vi "ESP_Full_State.vi"() -> ()   [LabVIEW 2021]
panel:
  in  "Channel":i32
  out "Data":dbl[](array[numeric])
  out "Stream on? UDP":string
  in  "file path 2":path
  in  "UDP Activate":bool
  out "All ESP":sgl[][](graph)
  in  "address":string="192.168.1.190"
  out "output array":sgl[][](array[numeric])
  in  "stop streaming":bool
  in  "Shut dowm":bool
  in  "Full state":bool
  in  "Stream":bool
  in  "Re-zero":bool
  out "Single ESP":sgl[](graph)
  out "Stream on?":string
  out "Full state on?":string
  out "Full state":string
  # "Sampling rate is 225 Hz, please use the Setup software to change the rate"
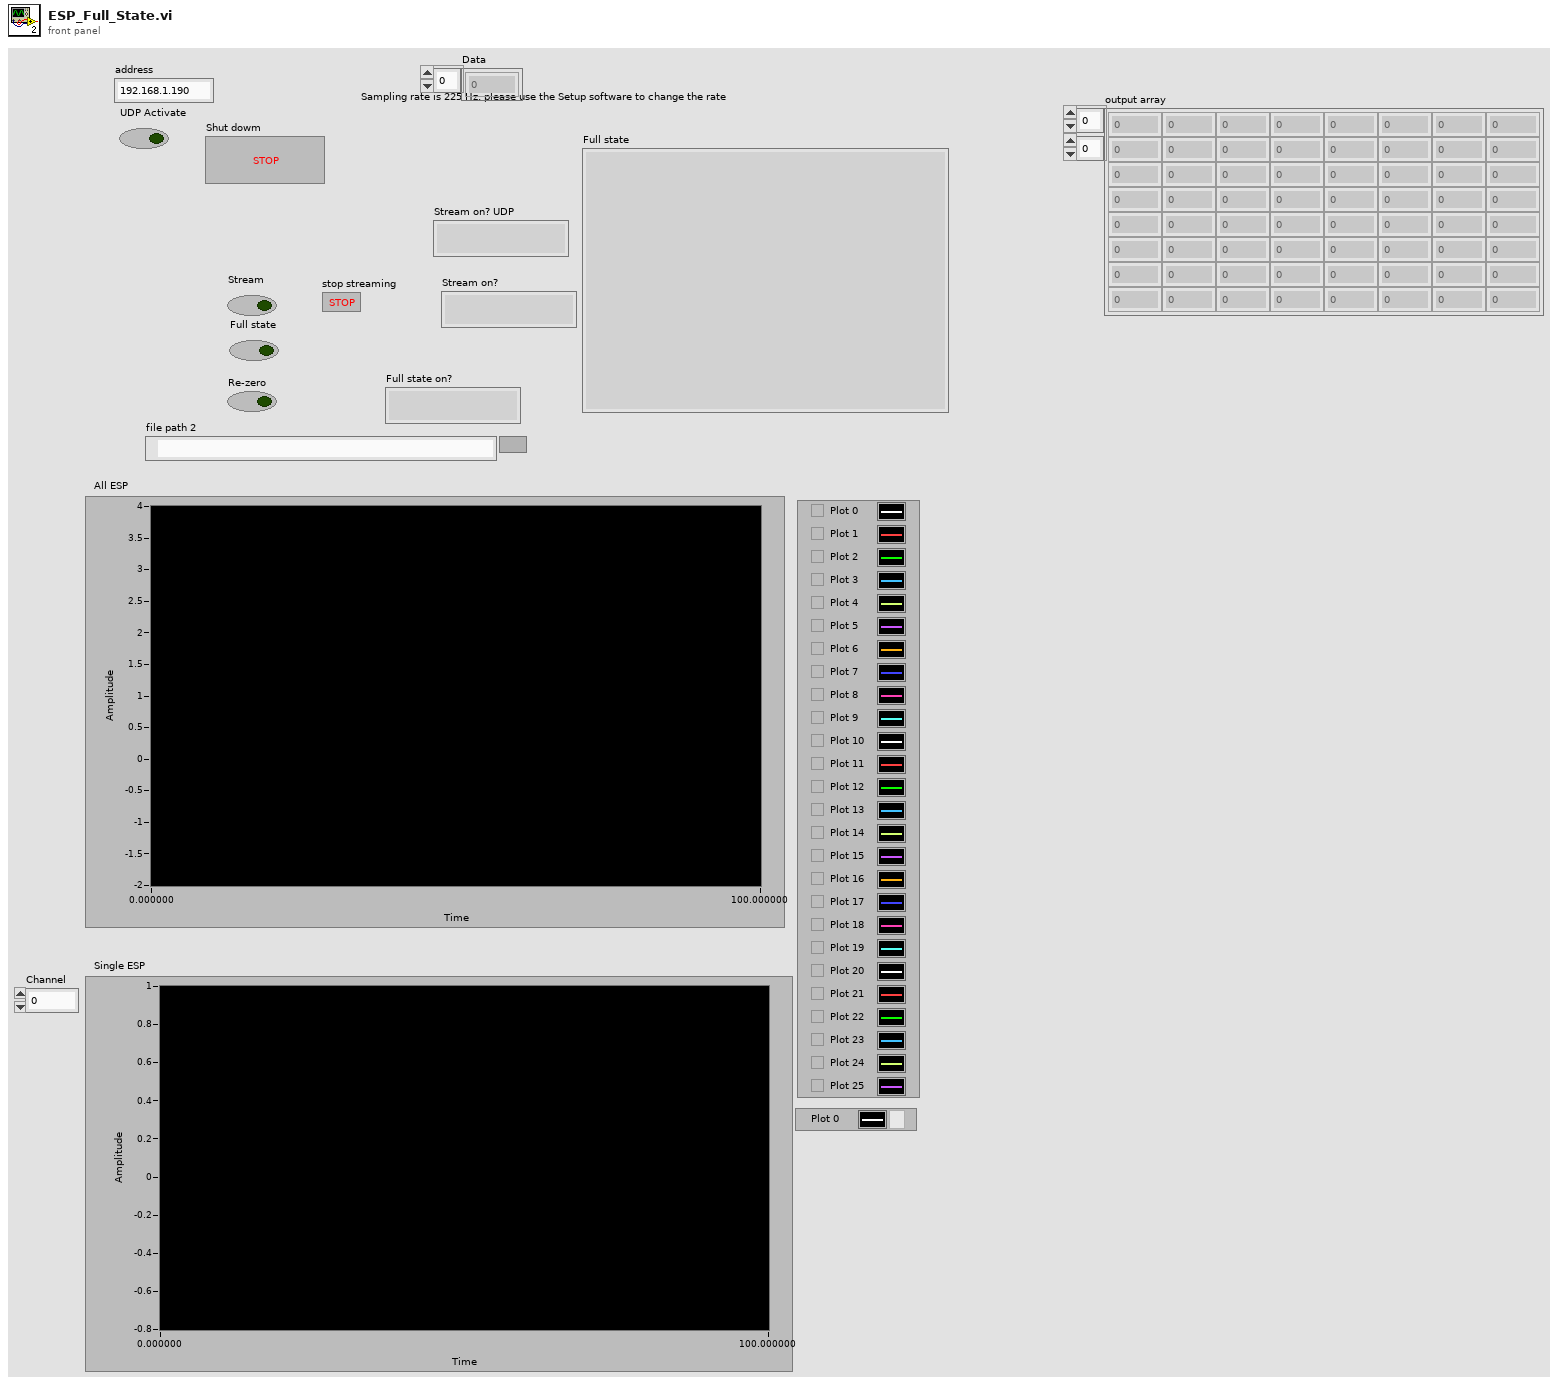
[diagram p1: front panel]
types:
  T1 = enum16{"Standard", "Buffered", "CRLF", "Immediate"}
  T2 = enum16{"open", "open or create", "create or replace", "create", "open (read-only)"}
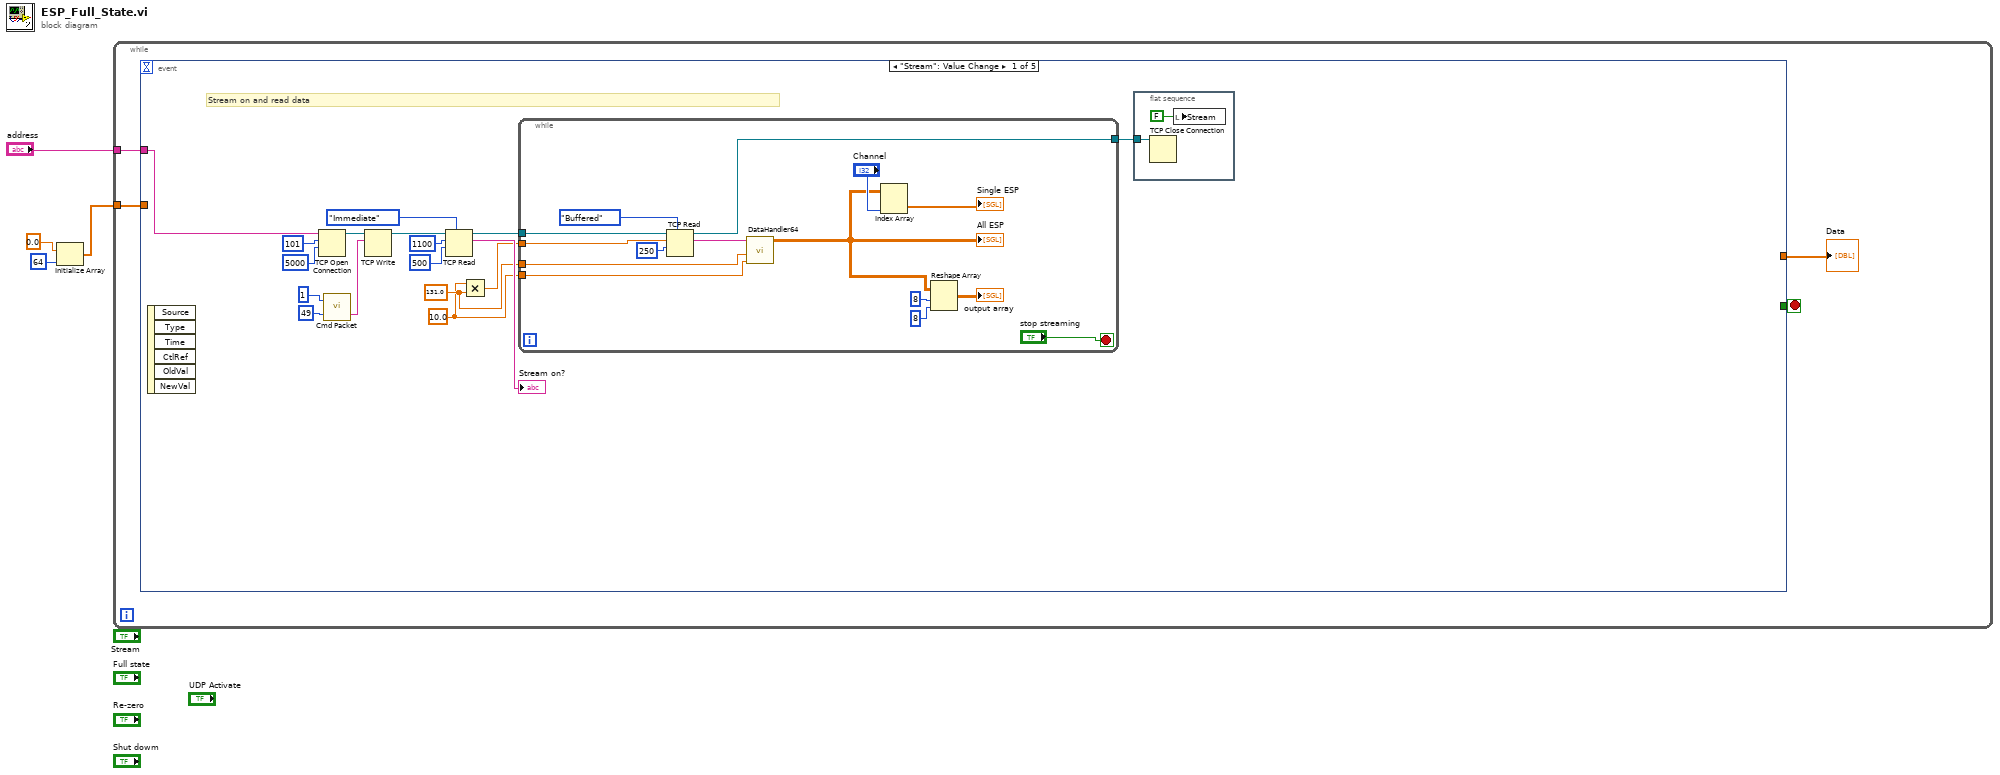
[diagram p0: block diagram]
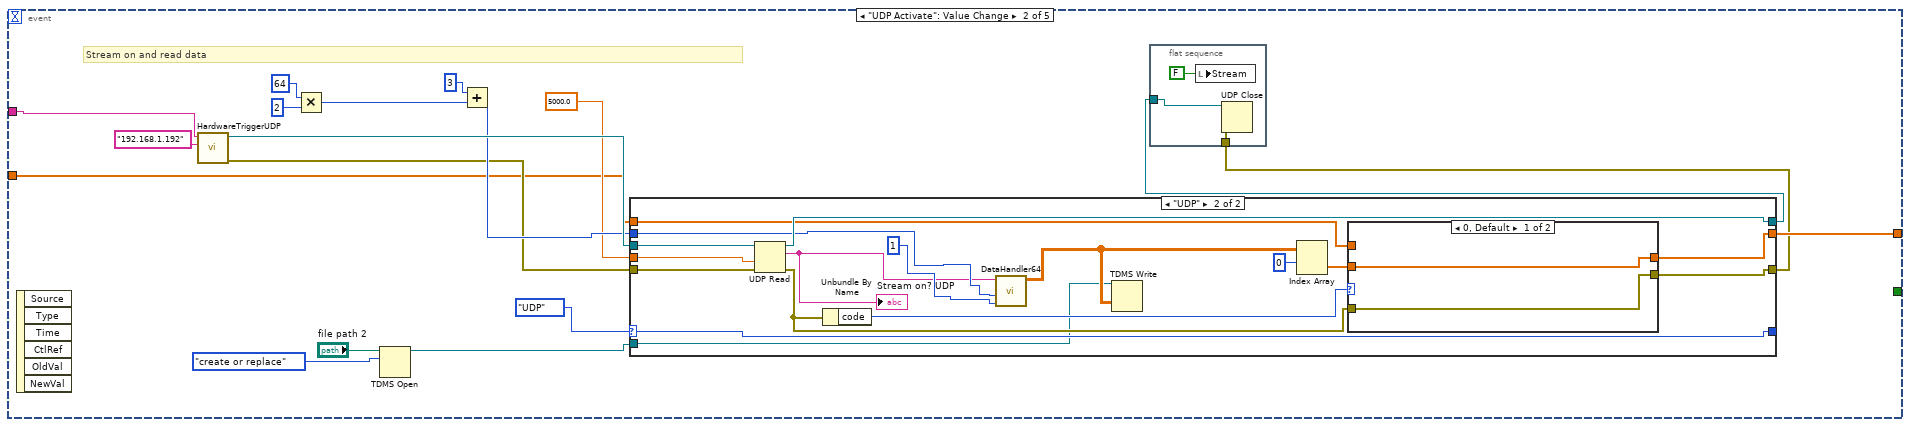
[diagram p2: hidden frame]
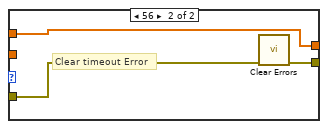
[diagram p4: hidden frame]
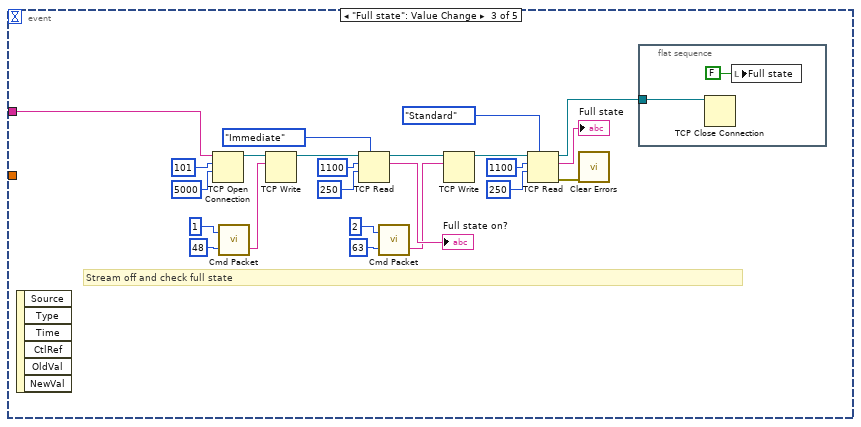
[diagram p5: hidden frame]
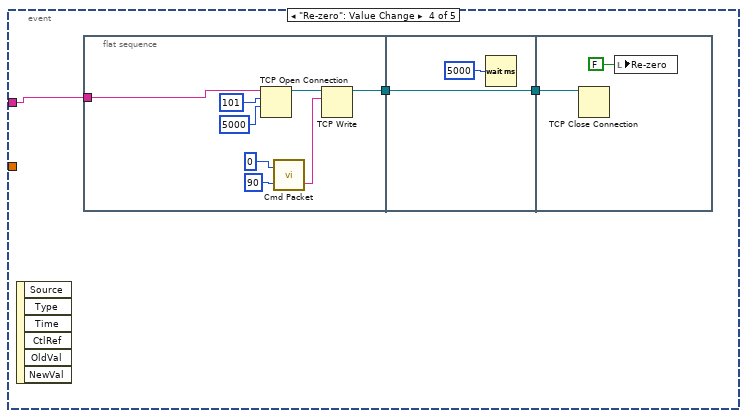
[diagram p6: hidden frame]
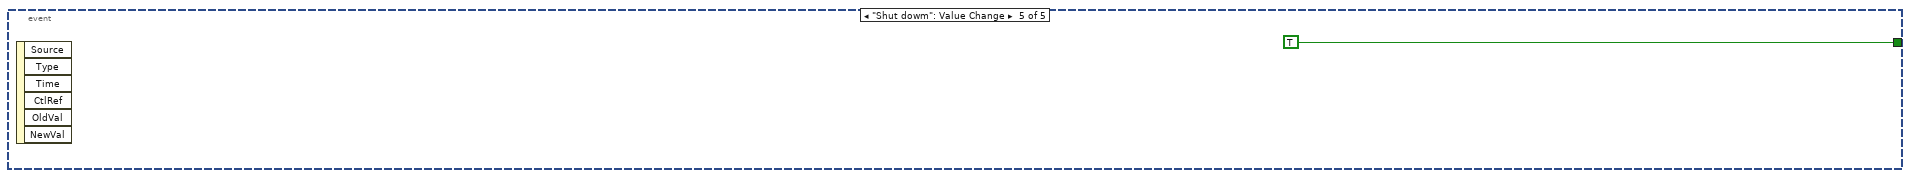
[diagram p7: hidden frame]
diagram:
  n1 = Initialize Array(0.0, 64) -> (w1:dbl[])
  n2 = while {
    tunnel: "address" -> [w7]
    tunnel: w1 -> [w6]
    stop <- w8 stop-if-true
    n3 = event shown="[0] \"Stream\": Value Change" {
      selector: _ -> [_ _ _ _ _]
      dyn-events: _ -> [_ _ _ _ _]
      timeout: _ -> [_ _ _ _ _]
      tunnel: [_ _ _ _ TRUE] -> w8
      tunnel: w7 -> [w9 w58 w90 w115 _]
      tunnel: w6 -> [_ w48 _ _ _]
      tunnel: [_ w44 _ _ _] -> w5
      event "Stream": Value Change {
        w10 = 10.0 ("Sampling Rate")
        w11 = 131.0 ("y")
        # "Stream on and read data"
        n4 = event-data() -> ()  [unwired: 1 in, 6 out]
        n5 = TCP Open Connection(address=w9, remote port or service name=u16 101 ("Port"), timeout ms (60000)=5000) -> (connection ID=w19:refnum<k5>)  [unwired: 2 in, 1 out]
        n6 = call "Cmd Packet.vi"("Command Byte"=49 ("data in"), "Parameter Byte"=1 ("data in")) -> ("Command Packet Byte String"=w23:string)  [unwired: 1 out]
        n7 = TCP Write(connection ID=w19, data in=w23) -> (connection ID out=w21:refnum<k5>)  [unwired: 2 in, 2 out]
        n8 = TCP Read(connection ID=w21, bytes to read=1100, 7:T1."Immediate" ("mode (standard)"), 9:500 ("timeout ms (25000)")) -> (connection ID out=w24:refnum<k5>, data out=→"Stream on?":string)  [unwired: 1 in, 1 out]
        n9 = Multiply(x=w10, y=w11) -> (x*y=w20:dbl)
        n10 = while {
          tunnel: [w39] -> w25
          tunnel: w24 -> [w35]
          tunnel: w20 -> [w38]
          tunnel: w11 -> [w37]
          tunnel: w10 -> [w36]
          stop <- "stop streaming" stop-if-true
          n11 = TCP Read(connection ID=w35, bytes to read=w38, 7:T1."Buffered" ("mode (standard)"), 9:250 ("timeout ms (25000)")) -> (connection ID out=w39:refnum<k5>, data out=w42:string)  [unwired: 1 in, 1 out]
          n12 = call "DataHandler64.vi"("Data Cycles Per Buffer"=w36, "Rx Packet Byte size"=w37, "data out"=w42) -> ("Data"=w28:sgl[][])  [unwired: 2 in, 4 out]
          "All ESP" <- w28
          n13 = Index Array(array=w28, index (col)="Channel") -> (element=→"Single ESP":sgl[])  [unwired: 1 in]
          n14 = Reshape Array(w28, 8 ("dimension size"), 8 ("dimension size")) -> (→"output array":sgl[][])
        }
        n15 = flat-sequence {
          tunnel: w25 -> [w26]
          frame #0 {
            n16 = TCP Close Connection(connection ID=w26) -> ()  [unwired: 2 in, 2 out]
            n17 = local write "Stream"(FALSE) -> ()
          }
        }
      }
      event "UDP Activate": Value Change {
        # "Stream on and read data"
        n18 = event-data() -> ()  [unwired: 1 in, 6 out]
        n19 = call "HardwareTriggerUDP.vi"("Local IP address"="192.168.1.192", "Remote IP address"=w58) -> ("error out"=w50:errorcluster, "connection ID out"=w56:refnum<k16>)  [unwired: 8 in]
        n20 = Multiply(x=64, y=2) -> (x*y=w54:i32)
        n21 = TDMS Open(10:T2."create or replace" ("operation (0:open)"), 11:"file path 2") -> (3:w46:refnum<k34>)  [unwired: 5 in, 1 out]
        n22 = Add(x=3, y=w54) -> (x+y=w51:i32)
        n23 = case shown="\"UDP\"" enum16{"Off", "UDP"}."UDP" {
          selector: enum16{"Off", "UDP"}."UDP" -> [w64 w80]
          tunnel: w51 -> [_ w68]
          tunnel: w50 -> [w63 w81]
          tunnel: [w63 w76] -> w43
          tunnel: [w64 w80] -> _
          tunnel: [w61 w72] -> w44
          tunnel: 5000.0 -> [_ w73]
          tunnel: w56 -> [w62 w75]
          tunnel: [w62 w74] -> w57
          tunnel: w48 -> [w61 w71]
          tunnel: w46 -> [_ w65]
          frame "Off", Default {
          }
          frame "UDP" {
            n24 = UDP Read(connection ID=w75, timeout ms (25000)=w73, 8:w81) -> (data out=w67:string, error out=w77:errorcluster, 3:w74:refnum<k16>)  [unwired: 1 in, 2 out]
            "Stream on? UDP" <- w67
            n25 = Unbundle By Name(w77) -> ("code"=w78:i32)
            n26 = call "DataHandler64.vi"("Data Cycles Per Buffer"=1, "Rx Packet Byte size"=w68, "data out"=w67) -> ("Data"=w66:sgl[][])  [unwired: 2 in, 4 out]
            n27 = TDMS Write(0:w65, 9:w66) -> ()  [unwired: 4 in, 4 out]
            n28 = Index Array(array=w66, index (row)=0 ("Data Cycles Per Buffer")) -> (element=w70:sgl[])  [unwired: 1 in]
            n29 = case shown="0, Default" w78 {
              tunnel: w77 -> [w83 w86]
              tunnel: [w83 w85] -> w76
              tunnel: w70 -> [w82 _]
              tunnel: [w82 w84] -> w72
              tunnel: w71 -> [_ w84]
              frame 0, Default {
              }
              frame 56 {
                # "Clear timeout Error"
                n30 = call <vilib>:"Clear Errors.vi"("error in (no error)"=w86) -> ("error out"=w85:errorcluster)  [unwired: 5 in, 1 out]
              }
            }
          }
        }
        n31 = flat-sequence {
          tunnel: w57 -> [w88]
          tunnel: w43 -> [w87]
          frame #0 {
            n32 = local write "Stream"(FALSE) -> ()
            n33 = UDP Close(connection ID=w88, 8:w87) -> ()  [unwired: 2 out]
          }
        }
      }
      event "Full state": Value Change {
        # "Stream off and check full state"
        n34 = event-data() -> ()  [unwired: 1 in, 6 out]
        n35 = TCP Open Connection(address=w90, remote port or service name=u16 101 ("Port"), timeout ms (60000)=5000) -> (connection ID=w92:refnum<k5>)  [unwired: 2 in, 1 out]
        n36 = call "Cmd Packet.vi"("Command Byte"=48 ("data in"), "Parameter Byte"=u32 1 ("element")) -> ("Command Packet Byte String"=w108:string)  [unwired: 1 out]
        n37 = TCP Write(connection ID=w92, data in=w108) -> (connection ID out=w111:refnum<k5>)  [unwired: 2 in, 2 out]
        n38 = TCP Read(connection ID=w111, bytes to read=1100, 7:T1."Immediate" ("mode (standard)"), 9:250 ("timeout ms (25000)")) -> (connection ID out=w112:refnum<k5>, data out=→"Full state on?":string)  [unwired: 1 in, 1 out]
        n39 = call "Cmd Packet.vi"("Command Byte"=63 ("data in"), "Parameter Byte"=2 ("data in")) -> ("Command Packet Byte String"=w105:string)  [unwired: 1 out]
        n40 = TCP Write(connection ID=w112, data in=w105) -> (connection ID out=w106:refnum<k5>)  [unwired: 2 in, 2 out]
        n41 = TCP Read(connection ID=w106, bytes to read=1100, 7:T1."Standard" ("mode (standard)"), 9:250 ("timeout ms (25000)")) -> (connection ID out=w91:refnum<k5>, data out=→"Full state":string, error out=w109:errorcluster)  [unwired: 1 in]
        n42 = call <vilib>:"Clear Errors.vi"("error in (no error)"=w109) -> ()  [unwired: 5 in, 2 out]
        n43 = flat-sequence {
          tunnel: w91 -> [w114]
          frame #0 {
            n44 = TCP Close Connection(connection ID=w114) -> ()  [unwired: 2 in, 2 out]
            n45 = local write "Full state"(FALSE ("Full state")) -> ()
          }
        }
      }
      event "Re-zero": Value Change {
        n46 = event-data() -> ()  [unwired: 1 in, 6 out]
        n47 = flat-sequence {
          tunnel: [w119] -> w116
          tunnel: w115 -> [w118]
          tunnel: [w127] -> w117
          tunnel: w116 -> [w127]
          tunnel: w117 -> [w128]
          frame #0 {
            n48 = TCP Open Connection(address=w118, remote port or service name=u16 101 ("Port"), timeout ms (60000)=5000) -> (connection ID=w125:refnum<k5>)  [unwired: 2 in, 1 out]
            n49 = call "Cmd Packet.vi"("Command Byte"=90 ("data in"), "Parameter Byte"=0 ("data in")) -> ("Command Packet Byte String"=w120:string)  [unwired: 1 out]
            n50 = TCP Write(connection ID=w125, data in=w120) -> (connection ID out=w119:refnum<k5>)  [unwired: 2 in, 2 out]
          }
          frame #1 {
            n51 = Wait (ms)(milliseconds to wait=u32 5000) -> ()  [unwired: 1 out]
          }
          frame #2 {
            n52 = TCP Close Connection(connection ID=w128) -> ()  [unwired: 2 in, 2 out]
            n53 = local write "Re-zero"(FALSE ("Re-zero")) -> ()
          }
        }
      }
      event "Shut dowm": Value Change {
        n54 = event-data() -> ()  [unwired: 1 in, 6 out]
      }
    }
    "Data" <- w5
  }
